vi "DashboardCell-Resize.vi"(6 "Cluster":T1={"Label Font Size"=24, "Data Font Size"=36, "String Font Size"=36}, 8 "error in (no error)":errorcluster, 9 "Cluster Size:Height":u32=134, 10 "Cluster Size:Width":u32=256, 11 "引气压力P4 4":refnum<vi>) -> (0 "error out":errorcluster, 1 "Bounds:Area Height":u32=134, 2 "Bounds:Area Width":u32=256)   [LabVIEW 2014, in "jkism-tool-support.lvlib"]
uses:
  jkism-tool-support.lvlib
panel:
  out "引气压力P4 2":T2={"Label"="Label", "Value"="0.00", "String"="0.00"} caption="Digital"
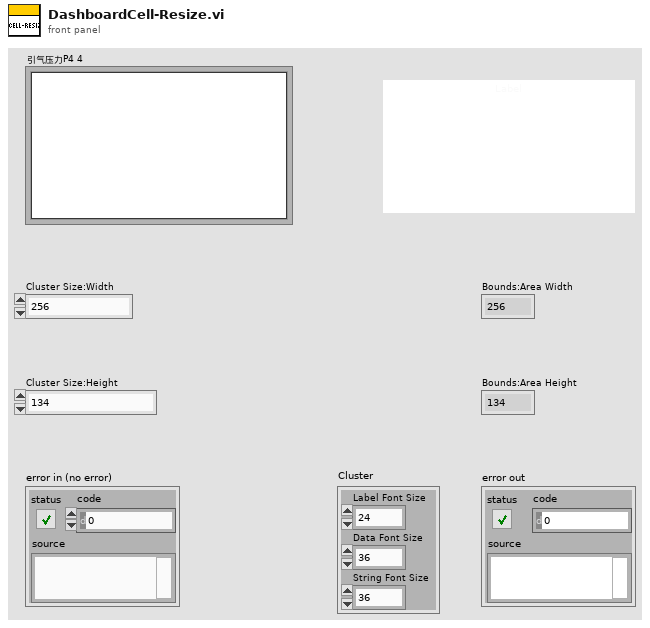
[diagram p1: front panel]
types:
  T1 = cluster{"Label Font Size":i32, "Data Font Size":i32, "String Font Size":i32}
  T2 = cluster{"Label":string, "Value":string, "String":string}
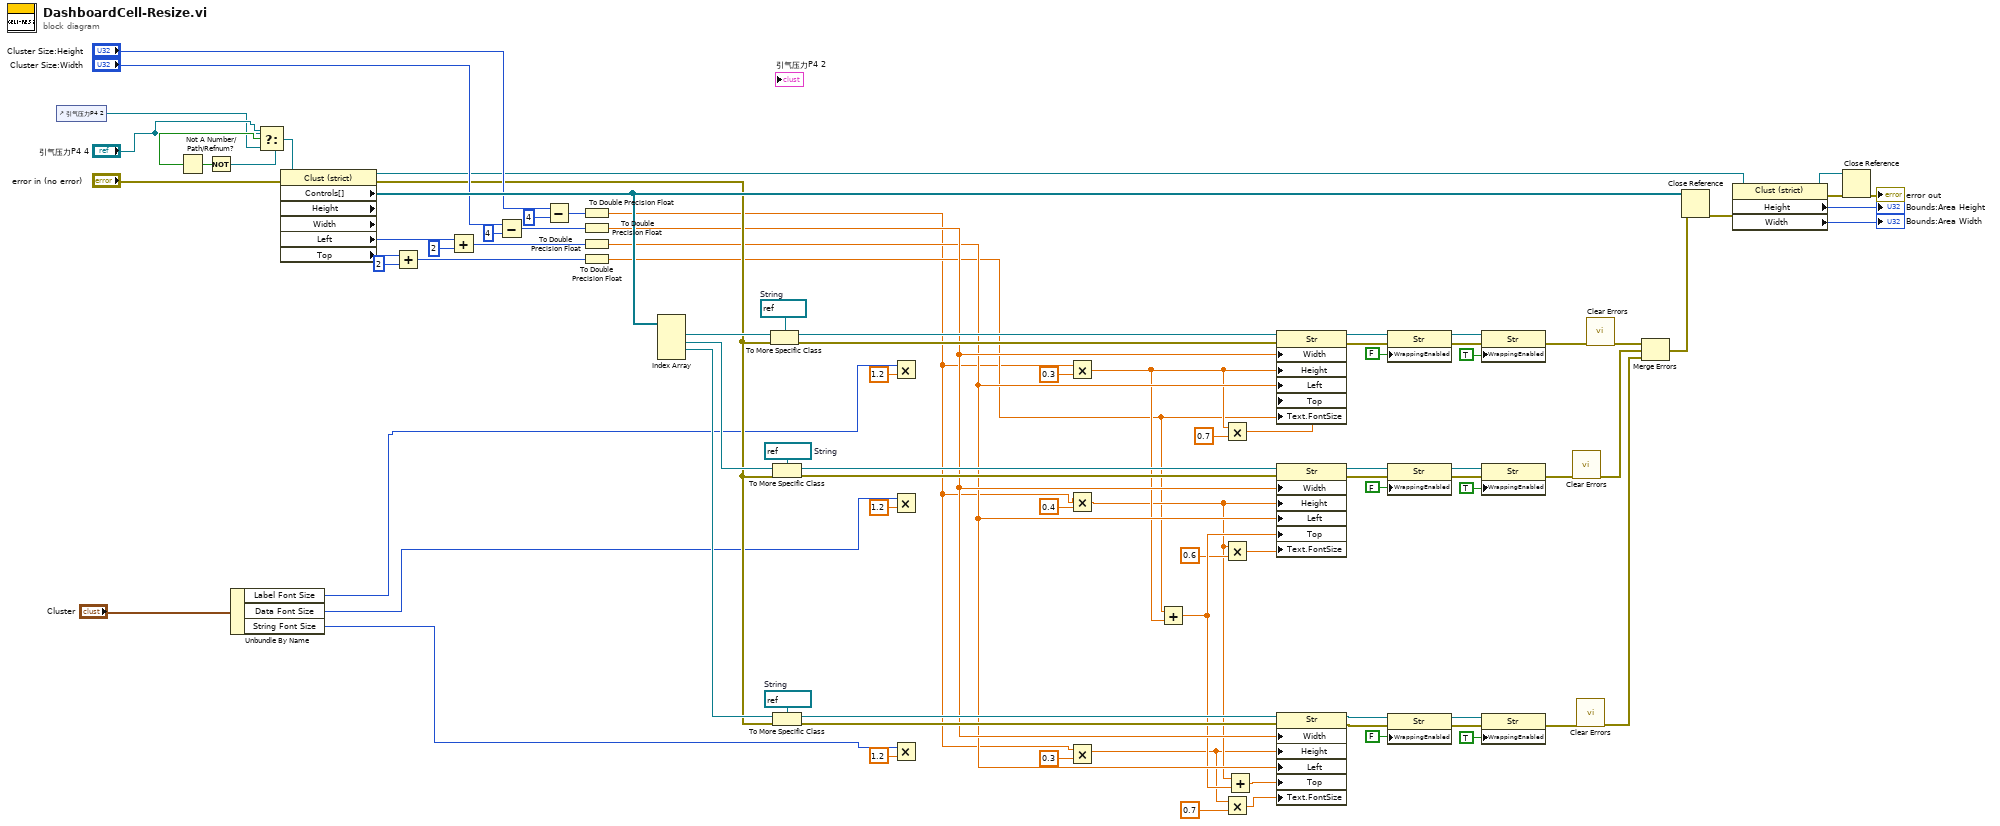
[diagram p0: block diagram]
diagram:
  w50 = refnum<vi> refnum  # String
  w84 = refnum<vi> refnum  # String
  w88 = refnum<vi> refnum  # String
  n1 = control-ref of="引气压力P4 2"() -> (w58:refnum<vi>)
  n2 = Not A Number/Path/Refnum?(number/path/refnum="引气压力P4 4") -> (NaN/Path/Refnum?=w1:bool)
  n3 = Not(x=w1) -> (.not. x?=w60:bool)
  n4 = Unbundle By Name("Cluster") -> ("Label Font Size"=w42:i32, "Data Font Size"=w41:i32, "String Font Size"=w40:i32)
  n5 = Select(t="引气压力P4 4", s=w60, f=w58) -> (s? t:f=w57:refnum<vi>)
  n6 = property on="Property Node" class="Clust (strict)" props=["Controls[]", "Height", "Width", "Left", "Top"](reference=w57, error in="error in (no error)") -> (reference out=w64:refnum<vi>, error out=w47:errorcluster, "Controls[]"=w89:refnum<vi>[], "Left"=w78:i32, "Top"=w75:i32)  [unwired: 2 out]
  n7 = Add(x=w75, y=2) -> (x+y=w54:i32)
  n8 = Add(x=w78, y=2) -> (x+y=w74:i32)
  n9 = Subtract(x="Cluster Size:Width", y=u32 4) -> (x-y=w81:u32)
  n10 = Subtract(x="Cluster Size:Height", y=u32 4) -> (x-y=w55:u32)
  n11 = To Double Precision Float(number=w55) -> (double precision float=w26:dbl)
  n12 = To Double Precision Float(number=w81) -> (double precision float=w46:dbl)
  n13 = To Double Precision Float(number=w74) -> (double precision float=w45:dbl)
  n14 = To Double Precision Float(number=w54) -> (double precision float=w30:dbl)
  n15 = Index Array(array=w89) -> (element #1=w86:refnum<vi>, element #2=w83:refnum<vi>, element #3=w48:refnum<vi>)  [unwired: 4 in, 1 out]
  n16 = To More Specific Class(target class=w88, reference=w86, error in=w47) -> (specific class reference=w87:refnum<vi>, error out=w70:errorcluster)
  n17 = To More Specific Class(target class=w84, reference=w83, error in=w47) -> (specific class reference=w85:refnum<vi>, error out=w71:errorcluster)
  n18 = To More Specific Class(target class=w50, reference=w48, error in=w47) -> (specific class reference=w49:refnum<vi>, error out=w51:errorcluster)
  n19 = Multiply(x=w42, y=1.2) -> ()  [unwired: 1 out]
  n20 = Multiply(x=w41, y=1.2) -> ()  [unwired: 1 out]
  n21 = Multiply(x=w40, y=1.2) -> ()  [unwired: 1 out]
  n22 = Multiply(x=w26, y=0.3) -> (x*y=w37:dbl)
  n23 = Multiply(x=w26, y=0.4) -> (x*y=w32:dbl)
  n24 = Multiply(x=w26, y=0.3) -> (x*y=w28:dbl)
  n25 = Add(x=w30, y=w37) -> (x+y=w44:dbl)
  n26 = Multiply(x=w37, y=0.7) -> (x*y=w38:dbl)
  n27 = Multiply(x=w32, y=0.6) -> (x*y=w33:dbl)
  n28 = Multiply(x=w28, y=0.7) -> (x*y=w29:dbl)
  n29 = Add(x=w32, y=w44) -> (x+y=w53:dbl)
  n30 = property on="Property Node" class="Str"(reference=w87, error in=w70, "Width"=w46, "Height"=w37, "Left"=w45, "Top"=w30, "Text.FontSize"=w38) -> (reference out=w22:refnum<vi>, error out=w21:errorcluster)
  n31 = property on="Property Node" class="Str"(reference=w85, error in=w71, "Width"=w46, "Height"=w32, "Left"=w45, "Top"=w44, "Text.FontSize"=w33) -> (reference out=w10:refnum<vi>, error out=w11:errorcluster)
  n32 = property on="Property Node" class="Str"(reference=w49, error in=w51, "Width"=w46, "Height"=w28, "Left"=w45, "Top"=w53, "Text.FontSize"=w29) -> (reference out=w4:refnum<vi>, error out=w3:errorcluster)
  n33 = property on="Property Node" class="Str"(reference=w22, error in=w21, "WrappingEnabled"=FALSE ("Enable Wrapping")) -> (reference out=w17:refnum<vi>, error out=w18:errorcluster)
  n34 = property on="Property Node" class="Str"(reference=w10, error in=w11, "WrappingEnabled"=FALSE ("Enable Wrapping")) -> (reference out=w15:refnum<vi>, error out=w14:errorcluster)
  n35 = property on="Property Node" class="Str"(reference=w4, error in=w3, "WrappingEnabled"=FALSE ("Enable Wrapping")) -> (reference out=w5:refnum<vi>, error out=w6:errorcluster)
  n36 = property on="Property Node" class="Str"(reference=w17, error in=w18, "WrappingEnabled"=TRUE ("Enable Wrapping")) -> (error out=w16:errorcluster)  [unwired: 1 out]
  n37 = property on="Property Node" class="Str"(reference=w15, error in=w14, "WrappingEnabled"=TRUE ("Enable Wrapping")) -> (error out=w9:errorcluster)  [unwired: 1 out]
  n38 = property on="Property Node" class="Str"(reference=w5, error in=w6, "WrappingEnabled"=TRUE ("Enable Wrapping")) -> (error out=w2:errorcluster)  [unwired: 1 out]
  n39 = call <vilib>:"Clear Errors.vi"("error in (no error)"=w9) -> ("error out"=w24:errorcluster)  [unwired: 6 in]
  n40 = call <vilib>:"Clear Errors.vi"("error in (no error)"=w2) -> ("error out"=w23:errorcluster)  [unwired: 6 in]
  n41 = call <vilib>:"Clear Errors.vi"("error in (no error)"=w16) -> ("error out"=w25:errorcluster)  [unwired: 6 in]
  n42 = Merge Errors(w25, w24, w23) -> (w82:errorcluster)
  n43 = Close Reference(reference=w89, error in (no error)=w82) -> (error out=w66:errorcluster)
  n44 = property on="Property Node" class="Clust (strict)"(reference=w64, error in=w66) -> (reference out=w63:refnum<vi>, error out=w65:errorcluster, "Height"=→"Bounds:Area Height":u32, "Width"=→"Bounds:Area Width":u32)
  n45 = Close Reference(reference=w63, error in (no error)=w65) -> (error out=→"error out":errorcluster)
